vi "HashPassword.vi"() -> ()   [LabVIEW 2025]
uses:
  <userlib>/_OpenG.lib/md5/md5.llb/MD5 Message Digest (Hexadecimal String)__ogtk.vi
panel:
  out "Hashed Password":string
  in  "Password":string
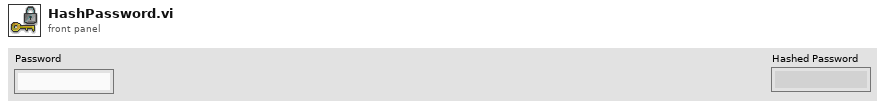
[diagram p1: front panel]
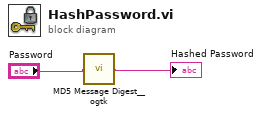
[diagram p0: block diagram]
diagram:
  n1 = call-poly <userlib>:"MD5 Message Digest__ogtk.vi"("Message"="Password") -> ("MD5 Message Digest"=→"Hashed Password":string)
